vi "Select Nodes In Rectangle.vi"(8 "error in (no error)":errorcluster, 9 "selectRect":T1, 11 "FSM in":refnum<class "FSM.Graph.lvclass">) -> (0 "error out":errorcluster, 3 "FSM out":refnum<class "FSM.Graph.lvclass">)   [LabVIEW 2020, in "FSM.Graph.lvclass"]
uses:
  FSM.Graph.lvclass
  FSM.Node/FSM.Node.lvclass
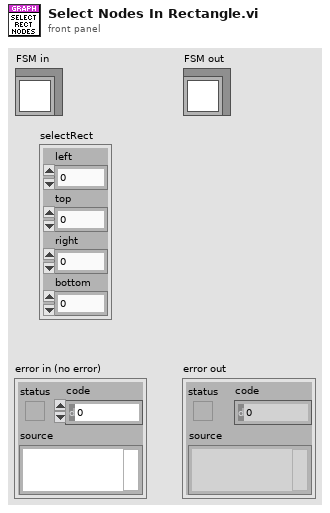
[diagram p1: front panel]
types:
  T1 = cluster{"left":i16, "top":i16, "right":i16, "bottom":i16}
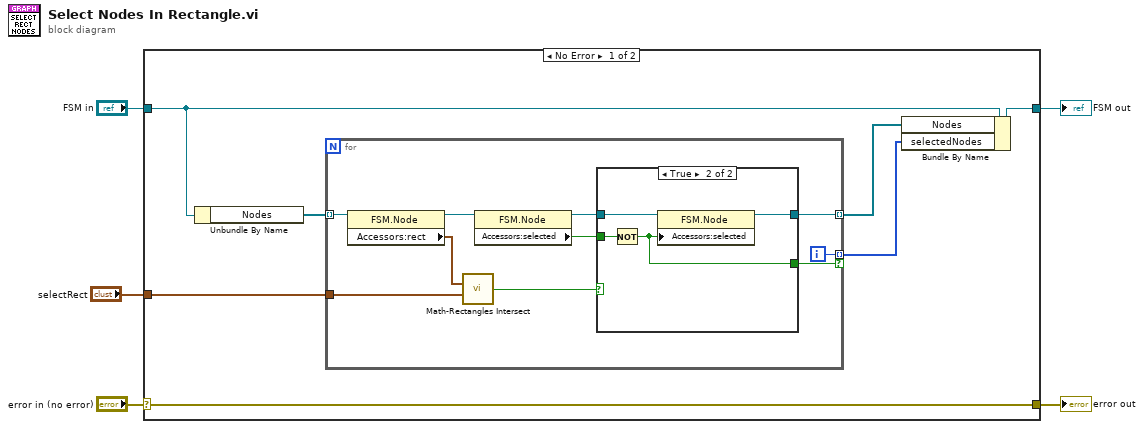
[diagram p0: block diagram]
diagram:
  n1 = case shown="No Error" "error in (no error)" {
    selector: "error in (no error)" -> [w12 w30]
    tunnel: [w12 w30] -> w4
    tunnel: [w9 w29] -> w2
    tunnel: "FSM in" -> [w11 w29]
    tunnel: "selectRect" -> [w6 _]
    frame No Error {
      n2 = Unbundle By Name(w11) -> ("Nodes"=w10:refnum<class "FSM.Node.lvclass">[])
      n3 = for {
        tunnel: w10 -> [w21] mode=indexing
        tunnel: [w22] -> w7 mode=indexing if=w16
        tunnel: [w17] -> w8 mode=indexing
        tunnel: w6 -> [w15]
        i -> [w22]
        n4 = property class="FSM.Node"(reference=w21) -> (reference out=w18:refnum<class "FSM.Node.lvclass">, "Accessors:rect"=w14:T1)  [unwired: 1 in, 1 out]
        n5 = call "Math-Rectangles Intersect.vi"("Rect1"=w14, "Rect2"=w15) -> ("intersect?"=w13:bool)  [unwired: 13 in]
        n6 = property class="FSM.Node"(reference=w18) -> (reference out=w19:refnum<class "FSM.Node.lvclass">, "Accessors:selected"=w20:bool)  [unwired: 1 in, 1 out]
        n7 = case shown="True" w13 {
          tunnel: w20 -> [w23 w28]
          tunnel: w19 -> [w24 w27]
          tunnel: [w24 w26] -> w17
          tunnel: [w23 w25] -> w16
          frame False {
          }
          frame True {
            n8 = Not(x=w28) -> (.not. x?=w25:bool)
            n9 = property class="FSM.Node"(reference=w27, "Accessors:selected"=w25) -> (reference out=w26:refnum<class "FSM.Node.lvclass">)  [unwired: 1 in, 1 out]
          }
        }
      }
      n10 = Bundle By Name(cluster=w11, "Nodes"=w8, "selectedNodes"=w7) -> (w9:refnum<class "FSM.Graph.lvclass">)
    }
    frame Error {
    }
  }
  "error out" <- w4
  "FSM out" <- w2
